vi "update disable settings.vi"(9 "disable":T1, 10 "channel index":i32, 11 "ZaberASeries in":refnum<class "ZaberASeries.lvclass">) -> (3 "ZaberASeries out":refnum<class "ZaberASeries.lvclass">)   [LabVIEW 2020, in "ZaberASeries.lvclass"]
uses:
  ZaberASeries.lvclass
  OnOffTypeDef.ctl
  ZaberASeries.lvclass/ZaberASeries.ctl
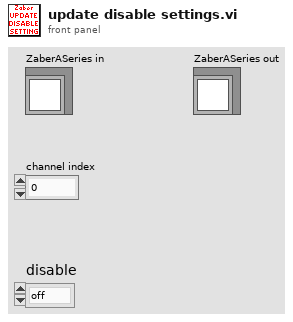
[diagram p1: front panel]
types:
  T1 = typedef "OnOffTypeDef.ctl" = enum16{"off", "on"}
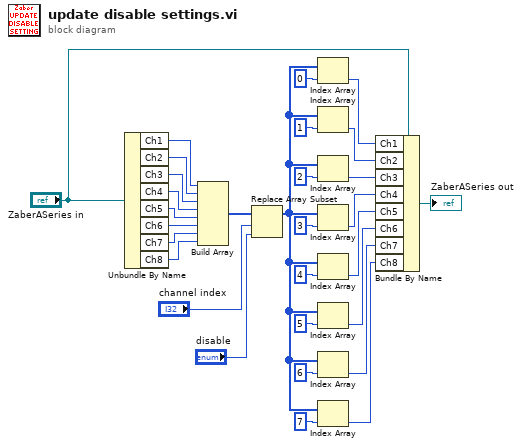
[diagram p0: block diagram]
diagram:
  n1 = Unbundle By Name("ZaberASeries in") -> ("Ch1"=w16:T1, "Ch2"=w17:T1, "Ch3"=w18:T1, "Ch4"=w19:T1, "Ch5"=w13:T1, "Ch6"=w12:T1, "Ch7"=w11:T1, "Ch8"=w10:T1)
  n2 = Build Array(w16, w17, w18, w19, w13, w12, w11, w10) -> (w20:T1[])
  n3 = Replace Array Subset(array=w20, new element="disable", index="channel index") -> (w5:T1[])
  n4 = Index Array(array=w5, index=0) -> (element=w27:T1)
  n5 = Index Array(array=w5, index=1) -> (element=w28:T1)
  n6 = Index Array(array=w5, index=2) -> (element=w30:T1)
  n7 = Index Array(array=w5, index=3) -> (element=w29:T1)
  n8 = Index Array(array=w5, index=4) -> (element=w4:T1)
  n9 = Index Array(array=w5, index=5) -> (element=w3:T1)
  n10 = Index Array(array=w5, index=6) -> (element=w2:T1)
  n11 = Index Array(array=w5, index=7) -> (element=w1:T1)
  n12 = Bundle By Name(cluster="ZaberASeries in", "Ch1"=w27, "Ch2"=w28, "Ch3"=w30, "Ch4"=w29, "Ch5"=w4, "Ch6"=w3, "Ch7"=w2, "Ch8"=w1) -> (→"ZaberASeries out":refnum<class "ZaberASeries.lvclass">)
